vi "Dc_transparency_test.vi"() -> ()   [LabVIEW 2013]
uses:
  <vilib>/DAQmx/read.llb/DAQmx Read (Analog 1D DBL 1Chan NSamp).vi
  <vilib>/DAQmx/read.llb/DAQmx Read (Analog DBL 1Chan 1Samp).vi
  <vilib>/DAQmx/create/channels.llb/DAQmx Create Channel (AI-Voltage-Basic).vi
  <vilib>/DAQmx/configure/timing.llb/DAQmx Timing (Sample Clock).vi
  <vilib>/DAQmx/miscellaneous.llb/DAQmx Fill In Error Info.vi
  <vilib>/Utility/file.llb/Write To Spreadsheet File (DBL).vi
  <resource>/objmgr/daqmx.rc
panel:
  in  "Concentration":dbl
  in  "LASER A/B":bool
  out "LASER B (continous)":dbl[](graph)
  out "LASER B (discrete)":dbl(graph)
  in  "Drop":dbl
  out "LASER A (continous)":dbl[](graph)
  out "Measurement File":path=path "C:/Users/Adam/Desktop/Diag_Prog_v9/testt"
  out "LASER A (discrete)":dbl(graph)
  in  "Ref channel":tag="Dev3/ai2"
  in  "stop":bool
  in  "Timer Start":bool
  in  "Start time":timestamp=timestamp(-9593251199.274853 s since 1904-01-01)
  in  "Record Button":bool
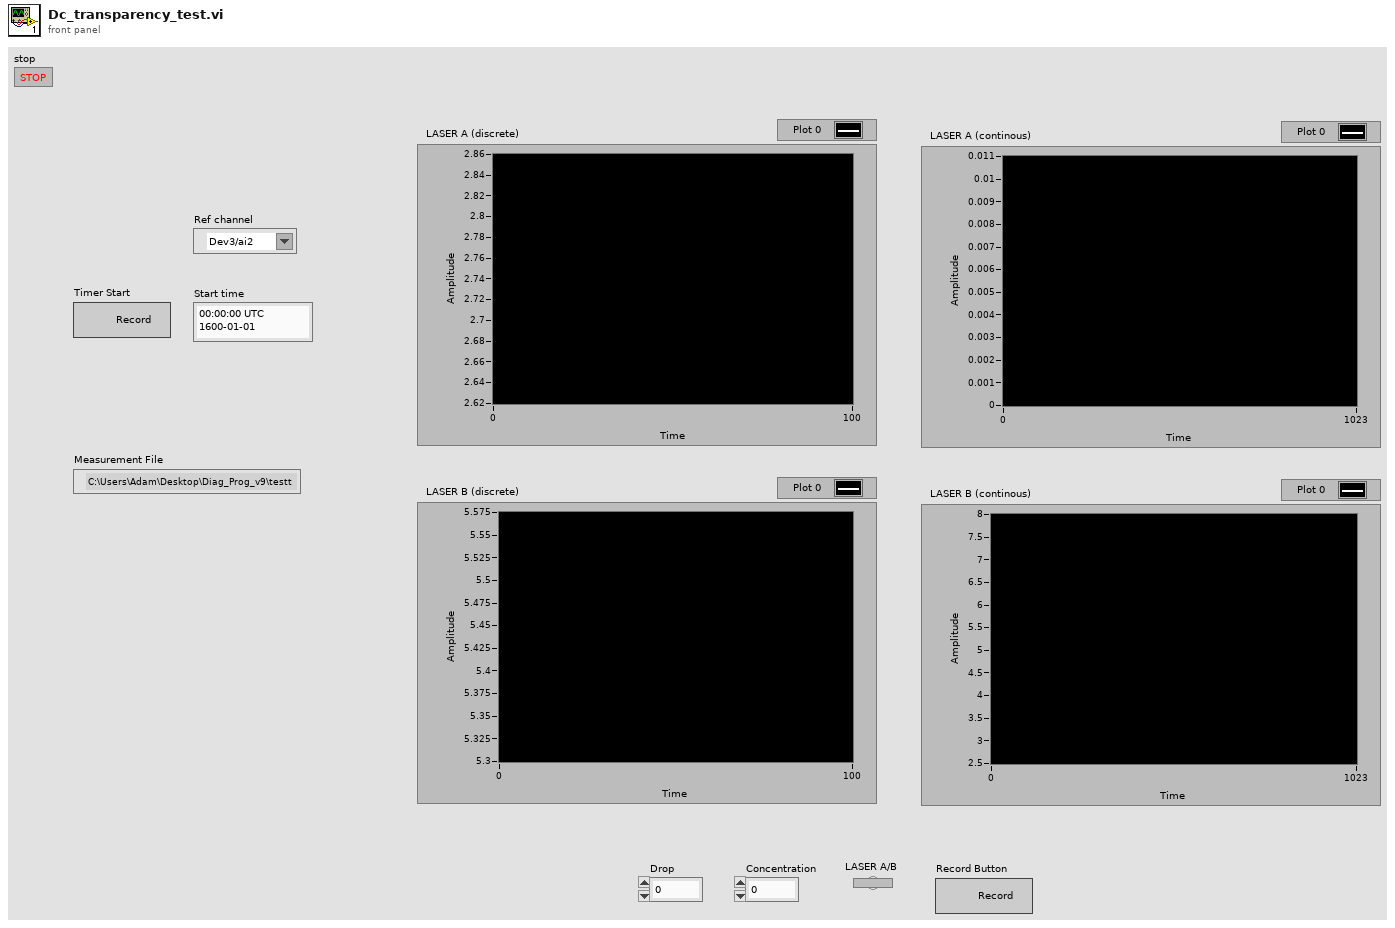
[diagram p1: front panel]
types:
  T1 = enum16{"open", "replace", "create", "open or create", "replace or create", "replace or create with confirmation"}
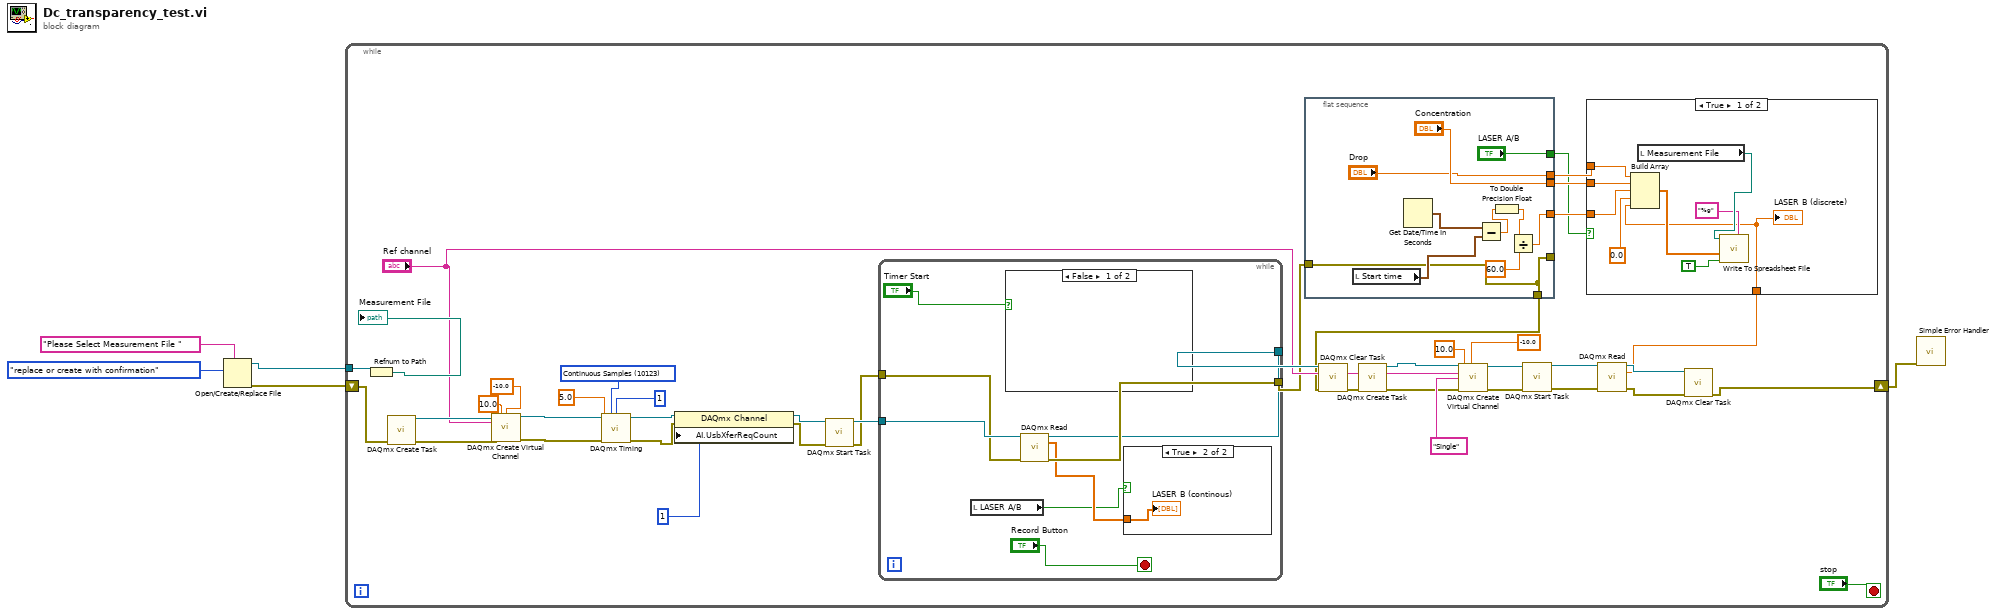
[diagram p0: block diagram]
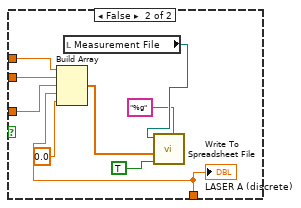
[diagram p2: hidden frame]
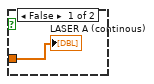
[diagram p3: hidden frame]
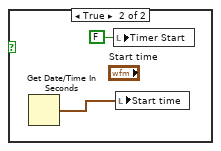
[diagram p4: hidden frame]
diagram:
  n1 = Open/Create/Replace File(prompt="Please Select Measurement File ", operation (0:open)=T1."replace or create with confirmation") -> (refnum out=w3:refnum<file>, error out=w2:errorcluster)  [unwired: 4 in, 1 out]
  n2 = while {
    tunnel: w3 -> [w46]
    shift-right: [w19] -> w1
    shift-left: w2 -> [w18]
    stop <- "stop" stop-if-true
    w22 = 10123 items=["Finite Samples"=10178, "Continuous Samples"=10123, "Hardware Timed Single Point"=12522] ("sample mode")
    n3 = Refnum to Path(1:w46) -> (0:→"Measurement File":path)
    n4 = call <vilib>:"DAQmx Create Task.vi"("error in"=w18) -> ("task out"=w21:refnum<k21>, "error out"=w20:errorcluster)  [unwired: 13 in]
    n5 = call-poly <vilib>:"DAQmx Create Virtual Channel.vi"("task in"=w21, "maximum value"=10.0, "minimum value"=-10.0, "physical channels"="Ref channel", "error in"=w20) -> ("task out"=w28:refnum<k21>, "error out"=w27:errorcluster)  [unwired: 9 in]
    n6 = call-poly <vilib>:"DAQmx Timing.vi"("task/channels in"=w28, "sample mode"=w22, "samples per channel"=1, "rate"=5.0, "error in"=w27) -> ("task out"=w23:refnum<k21>, "error out"=w24:errorcluster)  [unwired: 9 in]
    n7 = property class="DAQmx Channel"(reference=w23, error in=w24, "AI.UsbXferReqCount"=u32 1) -> (reference out=w17:refnum<k21>, error out=w16:errorcluster)
    n8 = call <vilib>:"DAQmx Start Task.vi"("task/channels in"=w17, "error in"=w16) -> ("task out"=w15:refnum<k21>, "error out"=w14:errorcluster)  [unwired: 12 in]
    n9 = while {
      tunnel: [w83] -> w8
      tunnel: [w81] -> w32
      tunnel: w15 -> [w80]
      tunnel: w14 -> [w79]
      stop <- "Record Button" stop-if-true
      n10 = local read "LASER A/B"() -> (w76:bool)
      n11 = case shown="False" "Timer Start" {
        frame False {
        }
        frame True {
          n12 = Get Date/Time In Seconds() -> (seconds since 1Jan1904=w87:timestamp)
          n13 = local write "Timer Start"(FALSE ("Timer Start")) -> ()
          n14 = local write "Start time"(w87) -> ()
        }
      }
      n15 = call-poly <vilib>:"DAQmx Read.vi"("task/channels in"=w80, "error in"=w79) -> ("task out"=w81:refnum<k21>, "data"=w77:dbl[], "error out"=w83:errorcluster)  [unwired: 11 in]
      n16 = case shown="True" w76 {
        tunnel: w77 -> [w84 w85]
        frame False {
          "LASER A (continous)" <- w84
        }
        frame True {
          "LASER B (continous)" <- w85
        }
      }
    }
    n17 = flat-sequence {
      tunnel: ["Concentration"] -> w12
      tunnel: ["Drop"] -> w11
      tunnel: [w50] -> w10
      tunnel: w8 -> [w49]
      tunnel: [w49] -> _
      tunnel: [w49] -> w7
      tunnel: ["LASER A/B"] -> w6
      frame #0 {
        n18 = local read "Start time"() -> (w53:timestamp)
        n19 = Get Date/Time In Seconds() -> (seconds since 1Jan1904=w57:timestamp)
        n20 = Subtract(x=w57, y=w53) -> (x-y=w55:dbl)
        n21 = To Double Precision Float(number=w55) -> (double precision float=w54:dbl)
        n22 = Divide(x=w54, y=60.0) -> (x/y=w50:dbl)
      }
    }
    n23 = call <vilib>:"DAQmx Clear Task.vi"("task in"=w32, "error in"=w7) -> ("error out"=w33:errorcluster)  [unwired: 13 in]
    n24 = call <vilib>:"DAQmx Create Task.vi"("error in"=w33) -> ("task out"=w41:refnum<k21>, "error out"=w40:errorcluster)  [unwired: 13 in]
    n25 = call-poly <vilib>:"DAQmx Create Virtual Channel.vi"("task in"=w41, "maximum value"=10.0, "minimum value"=-10.0, "physical channels"="Ref channel", "name to assign"="Single", "error in"=w40) -> ("task out"=w37:refnum<k21>, "error out"=w36:errorcluster)  [unwired: 8 in]
    n26 = call <vilib>:"DAQmx Start Task.vi"("task/channels in"=w37, "error in"=w36) -> ("task out"=w43:refnum<k21>, "error out"=w44:errorcluster)  [unwired: 12 in]
    n27 = call-poly <vilib>:"DAQmx Read.vi"("task/channels in"=w43, "error in"=w44) -> ("task out"=w34:refnum<k21>, "data"=w9:dbl, "error out"=w35:errorcluster)  [unwired: 11 in]
    n28 = case shown="True" w6 {
      tunnel: w9 -> [w58 w67]
      tunnel: w12 -> [w63 w72]
      tunnel: w11 -> [w62 w71]
      tunnel: w10 -> [w61 w70]
      frame True {
        n29 = Build Array(w62, w63, w61, 0.0 ("element"), w58) -> (w60:dbl[])
        n30 = local read "Measurement File"() -> (w66:path)
        n31 = call-poly <vilib>:"Write To Spreadsheet File.vi"("format (%.3f)"="%g", "append to file? (new file:F)"=TRUE, "1D data"=w60, "file path (dialog if empty)"=w66) -> ()  [unwired: 4 in, 1 out]
        "LASER B (discrete)" <- w58
      }
      frame False {
        n32 = Build Array(w71, w72, w70, w67, 0.0 ("element")) -> (w69:dbl[])
        n33 = local read "Measurement File"() -> (w75:path)
        n34 = call-poly <vilib>:"Write To Spreadsheet File.vi"("format (%.3f)"="%g", "append to file? (new file:F)"=TRUE, "1D data"=w69, "file path (dialog if empty)"=w75) -> ()  [unwired: 4 in, 1 out]
        "LASER A (discrete)" <- w67
      }
    }
    n35 = call <vilib>:"DAQmx Clear Task.vi"("task in"=w34, "error in"=w35) -> ("error out"=w19:errorcluster)  [unwired: 13 in]
  }
  n36 = call <vilib>:"Simple Error Handler.vi"("error in (no error)"=w1) -> ()  [unwired: 4 in, 5 out]
